vi "TestExec.Add Warning, Skip if redundant.vi"(9 "Warning":T1, 11 "Warning List":T1[](array[typedef])) -> (1 "Count":i32, 3 "Warning List Out":T1[](array[typedef]))   [LabVIEW 2018]
uses:
  Common/Utils/Errors/Error.Warning List Item.ctl
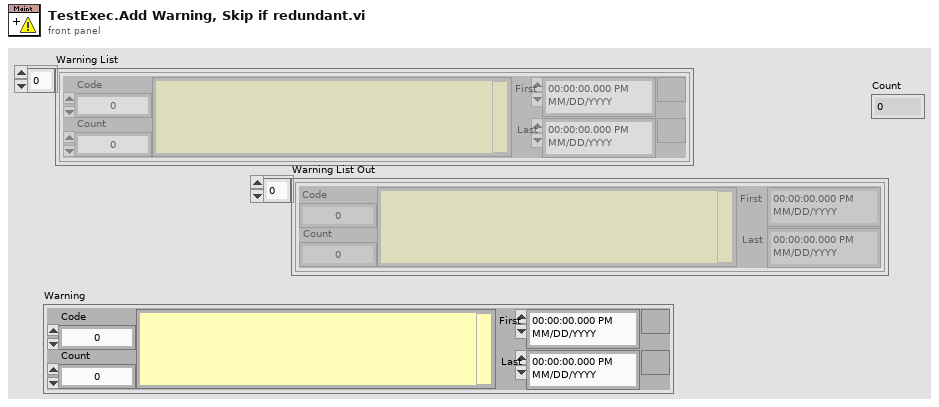
[diagram p1: front panel]
types:
  T1 = typedef "Error.Warning List Item.ctl" = cluster{"Code":i32, "Desc":string, "First":timestamp, "Last":timestamp, "Count":i32}
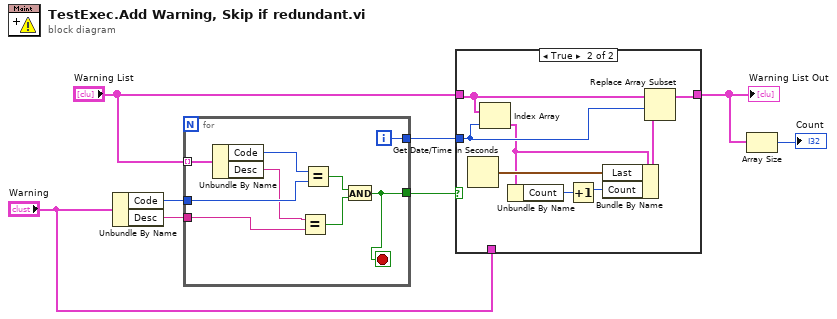
[diagram p0: block diagram]
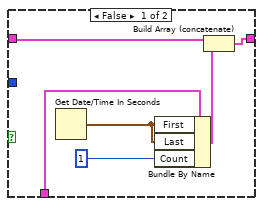
[diagram p2: hidden frame]
diagram:
  n1 = Unbundle By Name("Warning") -> ("Code"=w8:i32, "Desc"=w7:string)
  n2 = for {
    tunnel: "Warning List" -> [w17] mode=indexing
    tunnel: w8 -> [w13]
    tunnel: w7 -> [w11]
    tunnel: [w10] -> w6
    tunnel: [w9] -> w2
    i -> [w9]
    stop <- w10 stop-if-true
    n3 = Unbundle By Name(w17) -> ("Code"=w14:i32, "Desc"=w12:string)
    n4 = Equal?(x=w12, y=w11) -> (x = y?=w15:bool)
    n5 = Equal?(x=w14, y=w13) -> (x = y?=w16:bool)
    n6 = And(x=w16, y=w15) -> (x .and. y?=w10:bool)
  }
  n7 = case shown="True" w6 {
    tunnel: "Warning List" -> [w23 w28]
    tunnel: [w22 w31] -> w4
    tunnel: "Warning" -> [w21 _]
    tunnel: w2 -> [_ w29]
    frame False {
      n8 = Get Date/Time In Seconds() -> (seconds since 1Jan1904=w19:timestamp)
      n9 = Bundle By Name(cluster=w21, "First"=w19, "Last"=w19, "Count"=1) -> (w20:T1)
      n10 = Build Array (concatenate)(w23, w20) -> (w22:T1[])
    }
    frame True {
      n11 = Get Date/Time In Seconds() -> (seconds since 1Jan1904=w30:timestamp)
      n12 = Index Array(array=w28, index=w29) -> (element=w26:T1)
      n13 = Unbundle By Name(w26) -> ("Count"=w24:i32)
      n14 = Increment(x=w24) -> (x+1=w25:i32)
      n15 = Bundle By Name(cluster=w26, "Last"=w30, "Count"=w25) -> (w27:T1)
      n16 = Replace Array Subset(array=w28, new element=w27, index=w29) -> (w31:T1[])
    }
  }
  "Warning List Out" <- w4
  n17 = Array Size(array=w4) -> (size(s)=→"Count":i32)
